vi "Get IRQ.vi"(11 "IRQ":i32) -> (2 "function return":u32, 3 "IRQ out":i32)   [LabVIEW 2018, in "AndorSDK.lvlib"]
doc: "EXPNETTYPE unsigned int WINAPI GetIRQ(int * IRQ);"
uses:
  AndorSDK.lvlib
  ATMCD32D.dll
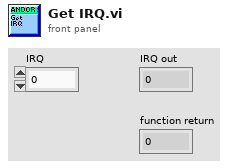
[diagram p1: front panel]
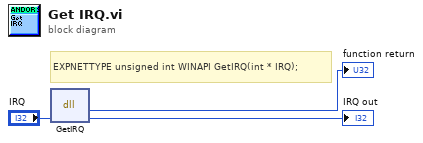
[diagram p0: block diagram]
diagram:
  # "EXPNETTYPE unsigned int WINAPI GetIRQ(int * IRQ);"
  n1 = dll-call lib="PTH2babs E\nPersönliches02 - Arbeit03-HiwijobsLabviewCodelibANDOR\tAndor SDK\nATMCD32D.*" fn="GetIRQ"("IRQ"="IRQ") -> (→"function return":u32, "IRQ"=→"IRQ out":i32)  [unwired: 3 in, 2 out]
